vi "Destination File Name.vi"(8 "Error In":errorcluster, 11 "File Stem":string) -> (0 "Error Out":errorcluster, 3 "Destination File Name":string)   [LabVIEW 2018, in "Scripts.lvlib"]
uses:
  Scripts.lvlib
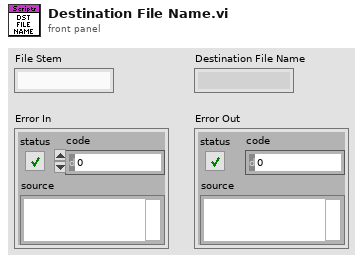
[diagram p1: front panel]
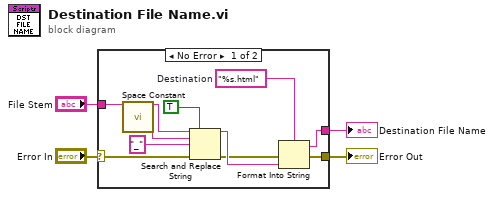
[diagram p0: block diagram]
diagram:
  n1 = case shown="No Error" "Error In" {
    selector: "Error In" -> [w6 w15]
    tunnel: "File Stem" -> [w11 _]
    tunnel: [w8 _] -> w3
    tunnel: [w7 w15] -> w2
    frame No Error {
      w9 = "%s.html"  # Destination
      n2 = call <vilib>:"Space Constant.vi"() -> ("String"=w13:string)
      n3 = Search and Replace String(replace all?=TRUE ("replace all? (F)"), input string=w11, search string=w13, replace string="_" ("replace string (\"\")"), error in=w6) -> (result string=w12:string, error out=w10:errorcluster)  [unwired: 3 in, 2 out]
      n4 = Format Into String(format string=w9, error in=w10, w12) -> (resulting string=w8:string, error out=w7:errorcluster)  [unwired: 1 in]
    }
    frame Error {
    }
  }
  "Destination File Name" <- w3
  "Error Out" <- w2
